vi "TIO Serial Port Name Search.vi"(10 "Default baud":i32=460800, 11 "String":string="serial:///dev/cu.usbserial-00000") -> (0 "Found port":bool=TRUE, 2 "Baud":i32=115200, 3 "VISA Resource":string="ASRL3::INSTR")   [LabVIEW 2019]
panel:
  out "Serial port string":string="/dev/cu.usbserial-00000"
  out "Resource List":string[](array[string])=["/dev/cu.Bluetooth-Incoming-Port", "", "/dev/cu.usbserial-00000"]
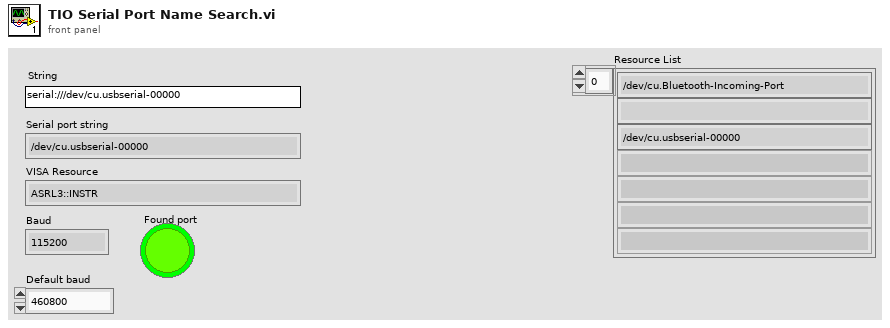
[diagram p1: front panel]
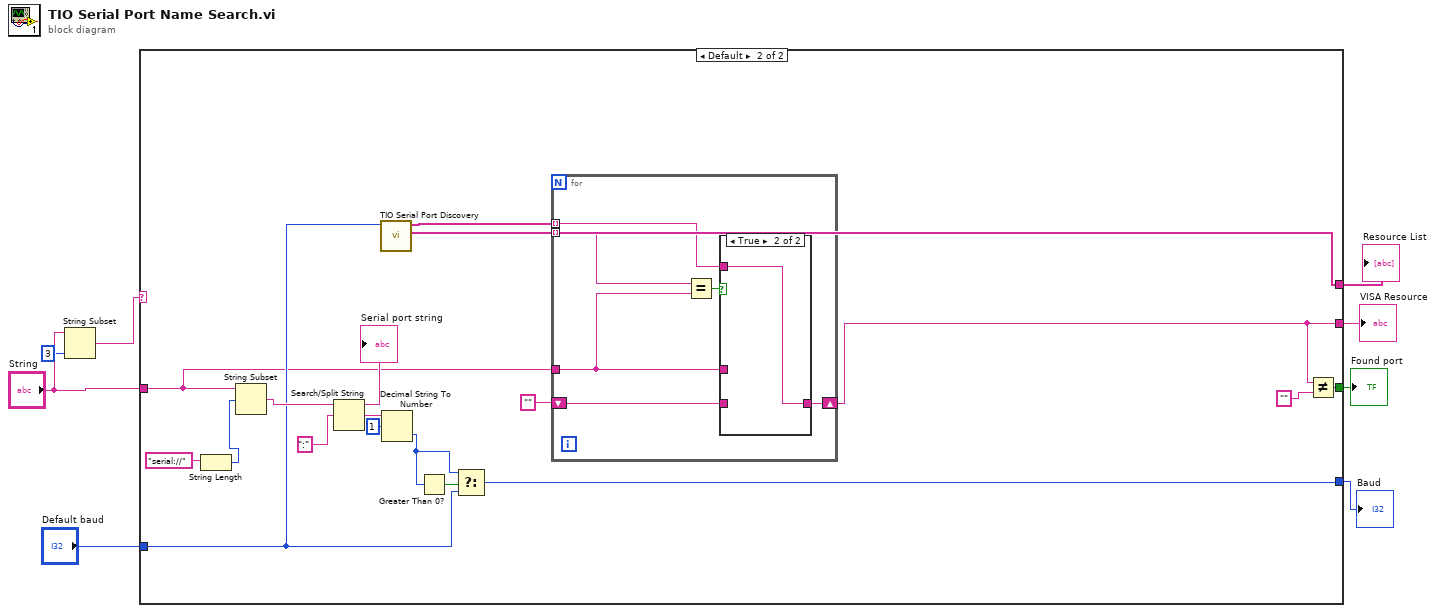
[diagram p0: block diagram]
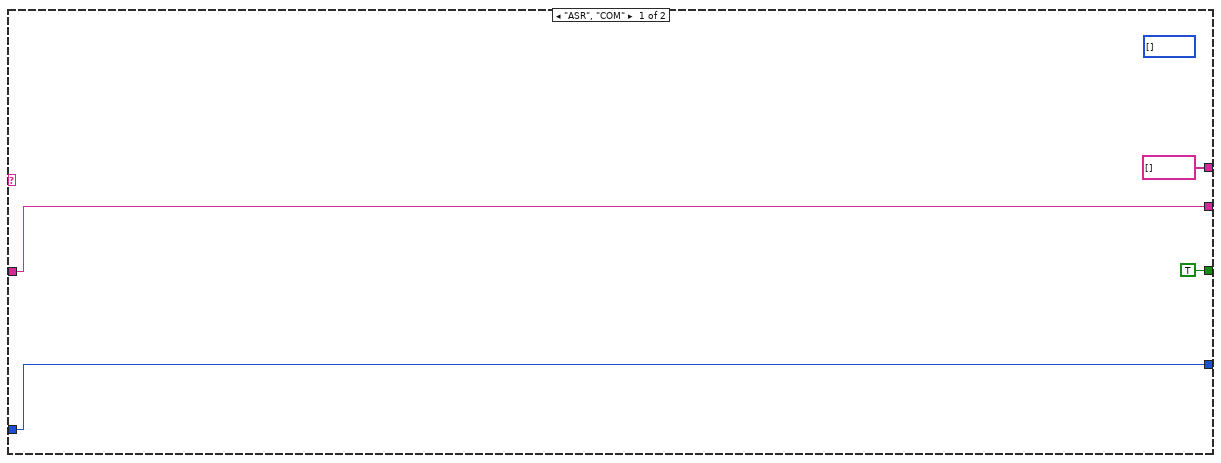
[diagram p2: hidden frame]
diagram:
  n1 = String Subset(string="String", length (rest)=3 ("length (rest)")) -> (substring=w4:string)  [unwired: 1 in]
  n2 = case shown="Default" w4 {
    tunnel: [string[] [] w17] -> w8
    tunnel: "String" -> [w12 w13]
    tunnel: [TRUE w21] -> w7
    tunnel: [w12 w15] -> w3
    tunnel: [w9 w20] -> w2
    tunnel: "Default baud" -> [w9 w18]
    frame "ASR", "COM" {
      (unwired) u16[] []
    }
    frame Default {
      n3 = String Length(string="serial://" ("search string/char (-)")) -> (length=w28:i32)
      n4 = String Subset(string=w13, offset (0)=w28) -> (substring=w27:string)  [unwired: 1 in]
      n5 = Search/Split String(string=w27, search string/char (-)=":") -> (substring before match=→"Serial port string":string, match + rest of string=w26:string)  [unwired: 1 in, 1 out]
      n6 = call "TIO Serial Port Discovery.vi"("Default baud"=w18) -> ("Device Names"=w17:string[], "VISA Names"=w14:string[])  [unwired: 9 in]
      n7 = Decimal String To Number(string=w26, offset=1) -> (number=w24:i32)  [unwired: 1 in, 1 out]
      n8 = Greater Than 0?(x=w24) -> (x > 0?=w23:bool)
      n9 = Select(t=w24, s=w23, f=w18) -> (s? t:f=w20:i32)
      n10 = for {
        tunnel: w17 -> [w36] mode=indexing
        tunnel: w13 -> [w32]
        shift-right: [w33] -> w15
        shift-left: "" -> [w35]
        tunnel: w14 -> [w31] mode=indexing
        n11 = Equal?(x=w36, y=w32) -> (x = y?=w34:bool)
        n12 = case shown="True" w34 {
          tunnel: w35 -> [w37 _]
          tunnel: [w37 w38] -> w33
          tunnel: w32 -> [_ _]
          tunnel: w31 -> [_ w38]
          frame False {
          }
          frame True {
          }
        }
      }
      n13 = Not Equal?(x=w15, y="") -> (x != y?=w21:bool)
    }
  }
  "Resource List" <- w8
  "Found port" <- w7
  "VISA Resource" <- w3
  "Baud" <- w2
